vi "Receive Initialization.vi"(8 "error in (no error)":errorcluster, 11 "Stream in":refnum<class "Stream.lvclass">) -> (0 "error out":errorcluster, 3 "Stream out":refnum<class "Stream.lvclass">)   [LabVIEW 2018, in "Stream.lvclass"]
uses:
  Stream.lvclass
  Stream.lvclass/Stream.ctl
  Interface/Interface.lvclass
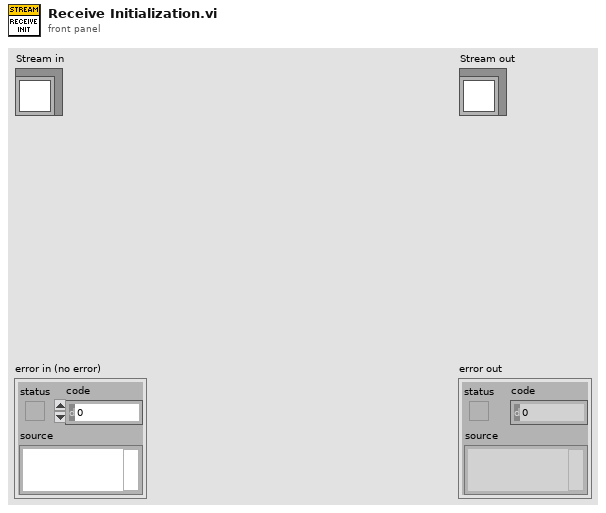
[diagram p1: front panel]
types:
  T1 = cluster{"Initialization":bool, "Serial Number":u16}
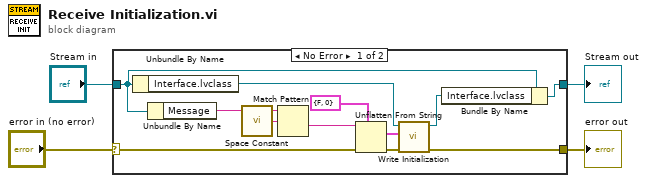
[diagram p0: block diagram]
diagram:
  n1 = case shown="No Error" "error in (no error)" {
    selector: "error in (no error)" -> [w16 w18]
    tunnel: [w8 w18] -> w2
    tunnel: [w12 w17] -> w1
    tunnel: "Stream in" -> [w11 w17]
    frame No Error {
      n2 = Unbundle By Name(w11) -> ("Interface.lvclass"=w10:refnum<class "Interface.lvclass">)
      n3 = Unbundle By Name(w11) -> ("Message"=w14:string)
      n4 = call <vilib>:"Space Constant.vi"() -> ("String"=w15:string)
      n5 = Match Pattern(string=w14, regular expression=w15) -> (after substring=w13:string)  [unwired: 1 in, 3 out]
      n6 = Unflatten From String(type=T1 {"Initialization"=FALSE, "Serial Number"=0} ("Initialization"), binary string=w13, error in (no error)=w16) -> (value=w6:T1, error out=w7:errorcluster)  [unwired: 2 in, 1 out]
      n7 = call "Write Initialization.vi"("error in (no error)"=w7, "Initialization"=w6, "Interface in"=w10) -> ("error out"=w8:errorcluster, "Interface out"=w9:refnum<class "Interface.lvclass">)  [unwired: 7 in]
      n8 = Bundle By Name(cluster=w11, "Interface.lvclass"=w9) -> (w12:refnum<class "Stream.lvclass">)
    }
    frame Error {
    }
  }
  "error out" <- w2
  "Stream out" <- w1
